vi "执行结果反馈与日志存储.vi"(9 "日志信息":string, 10 "error out":T1, 11 "设备":string) -> ()   [LabVIEW 2016]
panel:
  out "执行结果定义":u16(ring) items=["执行成功"=1, "执行失败，但不知道原因"=2, "命令请求条件错误"=3, "通讯超时"=4, "系统繁忙不能执行"=5, "系统故障"=6, "没有数据"=100]
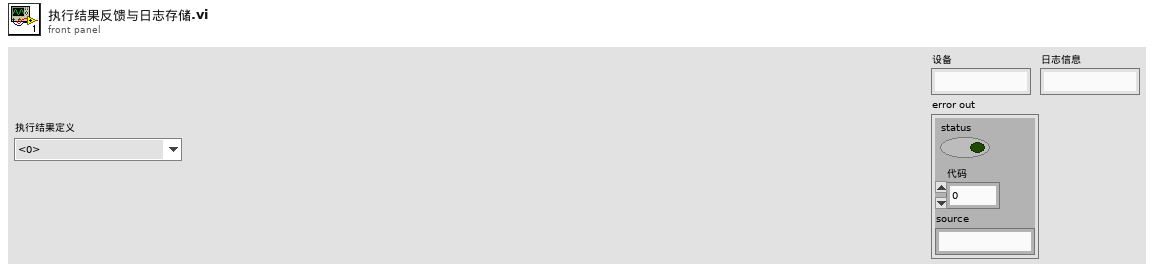
[diagram p1: front panel]
types:
  T1 = cluster{"status":bool, "代码":u16, "source":string}
  T2 = cluster{"时间标识":timestamp, "设备":string, "日志信息":string, "流程参数":string}
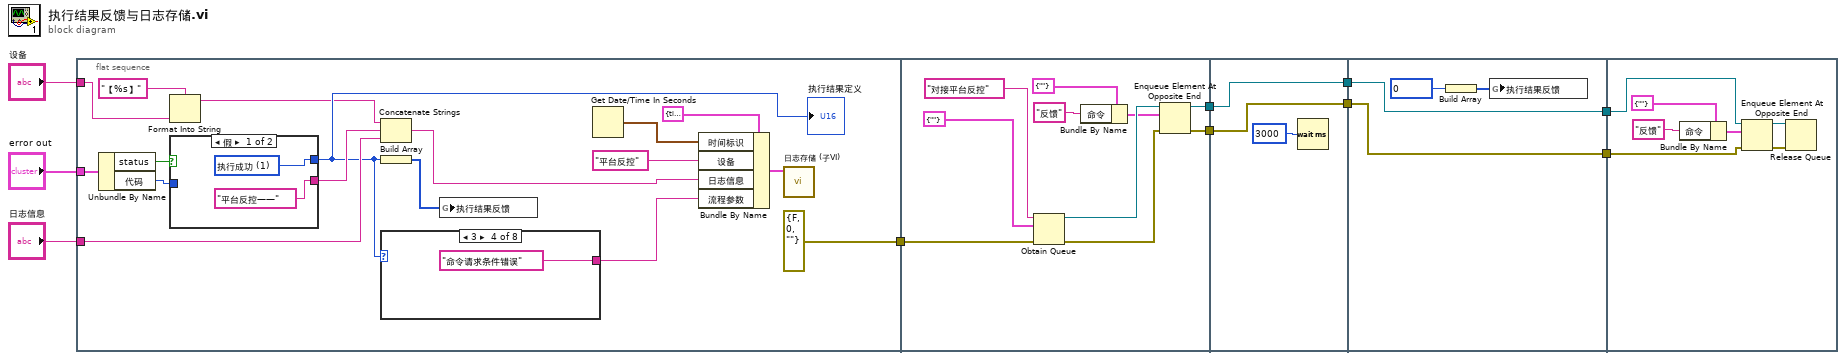
[diagram p0: block diagram]
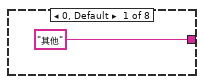
[diagram p2: hidden frame]
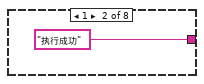
[diagram p3: hidden frame]
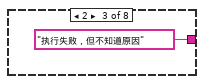
[diagram p4: hidden frame]
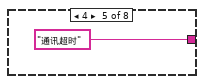
[diagram p5: hidden frame]
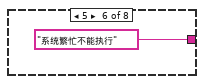
[diagram p6: hidden frame]
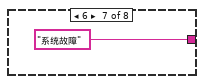
[diagram p7: hidden frame]
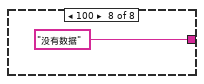
[diagram p8: hidden frame]
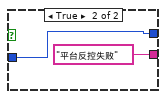
[diagram p9: hidden frame]
diagram:
  n1 = flat-sequence {
    tunnel: "日志信息" -> [w20]
    tunnel: "error out" -> [w19]
    tunnel: "设备" -> [w11]
    tunnel: [errorcluster {"status"=FALSE, "code"=0, "source"=""} ("错误输出")] -> w10
    tunnel: w10 -> [w42]
    tunnel: [w41] -> w9
    tunnel: [w40] -> w8
    tunnel: w9 -> [w52]
    tunnel: w8 -> [w51]
    tunnel: [w52] -> w7
    tunnel: [w51] -> w6
    tunnel: w7 -> [w54]
    tunnel: w6 -> [w53]
    tunnel: [w54] -> w5
    tunnel: [w53] -> w4
    tunnel: w5 -> [w60]
    tunnel: w4 -> [w59]
    frame #0 {
      n2 = Unbundle By Name(w19) -> ("status"=w26:bool, "代码"=w27:u16)
      n3 = Format Into String(format string="【%s】" ("格式字符串"), w11) -> (resulting string=w12:string)  [unwired: 2 in, 1 out]
      n4 = case shown="假" w26 {
        tunnel: ["平台反控——" ("日志信息") "平台反控失败" ("日志信息")] -> w25
        tunnel: [w36 w38] -> w16
        tunnel: w27 -> [_ w38]
        frame False {
          w36 = u16 1 items=["执行成功"=1, "执行失败，但不知道原因"=2, "命令请求条件错误"=3, "通讯超时"=4, "系统繁忙不能执行"=5, "系统故障"=6, "没有数据"=100] ("执行结果定义")
        }
        frame True {
        }
      }
      "执行结果定义" <- w16
      n5 = Concatenate Strings(w12, w25, w20) -> (w24:string)
      n6 = Build Array(w16) -> (w18:u16[])
      n7 = case shown="3" w16 {
        tunnel: ["其他" "执行成功" "执行失败，但不知道原因" "命令请求条件错误" "通讯超时" "系统繁忙不能执行" "系统故障" "没有数据"] -> w15
        frame 0, Default {
        }
        frame 1 {
        }
        frame 2 {
        }
        frame 3 {
        }
        frame 4 {
        }
        frame 5 {
        }
        frame 6 {
        }
        frame 100 {
        }
      }
      n8 = global write "modbus slave全局.vi" "执行结果反馈"(w18) -> ()
      n9 = Get Date/Time In Seconds() -> (seconds since 1Jan1904=w21:timestamp)
      n10 = Bundle By Name(cluster=T2 {"时间标识"=timestamp(0 s since 1904-01-01), "设备"="", "日志信息"="", "流程参数"=""} ("data in"), "时间标识"=w21, "设备"="平台反控", "日志信息"=w24, "流程参数"=w15) -> (w22:T2)
      n11 = call "日志存储 (子VI).vi"("data in"=w22) -> ()  [unwired: 11 in]
    }
    frame #1 {
      n12 = Obtain Queue(name (unnamed)="对接平台反控" ("名称（未命名）"), element data type=cluster{"命令":string} {"命令"=""}, error in (no error)=w42) -> (queue out=w47:refnum<queue>, error out=w46:errorcluster)  [unwired: 2 in, 1 out]
      n13 = Bundle By Name(cluster=cluster{"命令":string} {"命令"=""} ("元素"), "命令"="反馈") -> (w43:cluster{"命令":string})
      n14 = Enqueue Element At Opposite End(queue=w47, element=w43, error in (no error)=w46) -> (queue out=w41:refnum<queue>, error out=w40:errorcluster)  [unwired: 1 in, 1 out]
    }
    frame #2 {
      n15 = Wait (ms)(milliseconds to wait=u32 3000 ("等待时间（毫秒）")) -> ()  [unwired: 1 out]
    }
    frame #3 {
      w55 = u16 0 items=["执行成功"=1, "执行失败，但不知道原因"=2, "命令请求条件错误"=3, "通讯超时"=4, "系统繁忙不能执行"=5, "系统故障"=6, "没有数据"=100] ("执行结果定义")
      n16 = Build Array(w55) -> (w56:u16[])
      n17 = global write "modbus slave全局.vi" "执行结果反馈"(w56) -> ()
    }
    frame #4 {
      n18 = Bundle By Name(cluster=cluster{"命令":string} {"命令"=""} ("元素"), "命令"="反馈") -> (w61:cluster{"命令":string})
      n19 = Enqueue Element At Opposite End(queue=w60, element=w61, error in (no error)=w59) -> (queue out=w58:refnum<queue>, error out=w57:errorcluster)  [unwired: 1 in, 1 out]
      n20 = Release Queue(queue=w58, error in (no error)=w57) -> ()  [unwired: 1 in, 3 out]
    }
  }
